vi "Write Scrubbers.vi"(8 "error in":errorcluster, 10 "Scrubbers":refnum<class "Scrubber.lvclass">[](array[class]), 11 "Multi Scrubber in":refnum<class "Multi Scrubber.lvclass">) -> (0 "error out":errorcluster, 3 "Multi Scrubber out":refnum<class "Multi Scrubber.lvclass">)   [LabVIEW 2020, in "Approval Tests.lvlib" / "Multi Scrubber.lvclass"]
uses:
  Multi Scrubber.lvclass
  Scrubber/Scrubber.lvclass
  Multi Scrubber.lvclass/Multi Scrubber.ctl
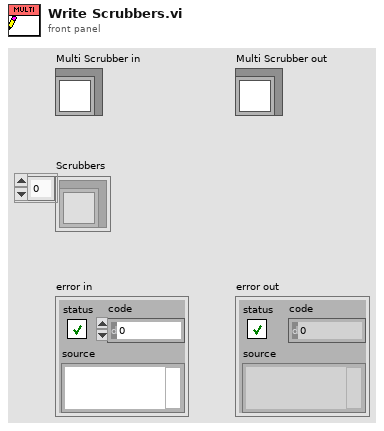
[diagram p1: front panel]
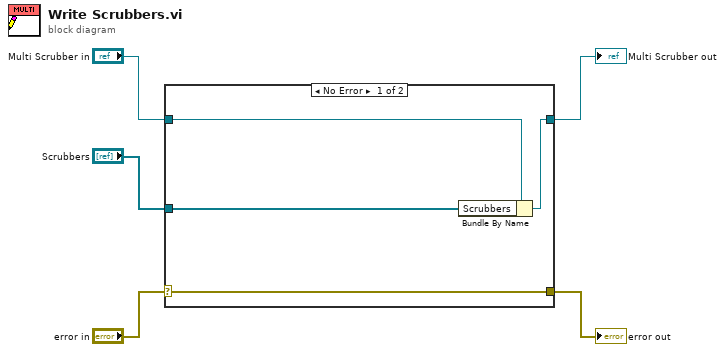
[diagram p0: block diagram]
diagram:
  n1 = case shown="No Error" "error in" {
    selector: "error in" -> [w9 w11]
    tunnel: [w9 w11] -> w4
    tunnel: [w7 w10] -> w2
    tunnel: "Multi Scrubber in" -> [w8 w10]
    tunnel: "Scrubbers" -> [w6 _]
    frame No Error {
      n2 = Bundle By Name(cluster=w8, "Scrubbers"=w6) -> (w7:refnum<class "Multi Scrubber.lvclass">)
    }
    frame Error {
    }
  }
  "error out" <- w4
  "Multi Scrubber out" <- w2
